vi "Init.vi"(8 "error in":errorcluster, 10 "<JSON> Scaling Config":string, 11 "Scalar Scaling Strategy in":refnum<class "Scalar Scaling Strategy.lvclass">) -> (0 "error out":errorcluster, 3 "Scalar Scaling Strategy out":refnum<class "Scalar Scaling Strategy.lvclass">)   [LabVIEW 2024, in "HAL.lvlib" / "Scalar Scaling Strategy.lvclass"]
uses:
  Scalar Scaling Strategy.lvclass
  Scalar Scaling Strategy.lvclass/Scalar Scaling Strategy.ctl
  394e7266-cc86-4bad-be5e-31de06d759fb.vi
  <vilib>/JDP Science/JSONtext/JSON text to Variant.vi
  <vilib>/JDP Science/JSONtext/LVClass Serializer/JSONtext LVClass Serializer.lvclass
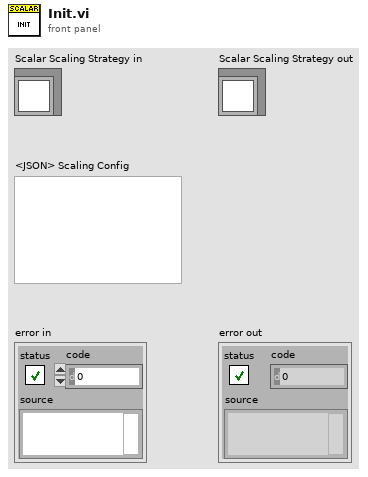
[diagram p1: front panel]
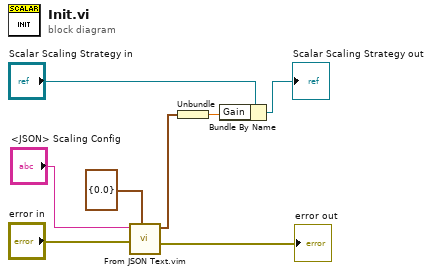
[diagram p0: block diagram]
diagram:
  n1 = call "From JSON Text.vim"("Data Type and Default Value"=cluster{"Gain":dbl} {"Gain"=0.0}, "error in (no error)"="error in", "JSON"="<JSON> Scaling Config") -> ("error out"=→"error out":errorcluster, "Data out"=w2:cluster{"Gain":dbl})  [unwired: 7 in]
  n2 = Unbundle(w2) -> ("Gain"=w1:dbl)
  n3 = Bundle By Name(cluster="Scalar Scaling Strategy in", "Gain"=w1) -> (→"Scalar Scaling Strategy out":refnum<class "Scalar Scaling Strategy.lvclass">)
